vi "Process.vi"(8 "error in (no error)":errorcluster, 10 "Pound in":refnum<class "Pound.lvclass">, 11 "Qbus in":refnum<class "Qbus.lvclass">) -> (0 "error out":errorcluster)   [LabVIEW 2017, in "EmsaAnalysis.lvlib"]
uses:
  <vilib>/addons/InsightCM/Devices/Shared/Emsa/EmsaAnalysis/EmsaAnalysis.lvlib
  <vilib>/addons/Qbus/Qbus.lvclass
  <vilib>/NI/Software Watchdog/Pound/Pound.lvclass
  <vilib>/addons/InsightCM/Devices/Shared/Emsa/EmsaAnalysis/controls/datagroupMetrics.ctl
  <vilib>/addons/InsightCM/Devices/Shared/Emsa/EmsaAnalysis/controls/channelMetrics.ctl
  <vilib>/addons/InsightCM/Devices/Shared/Emsa/EmsaAnalysis/controls/metric.ctl
  <vilib>/addons/InsightCM/MessageBus/Base/controls/MetricDefinitionInstance.ctl
  <vilib>/addons/InsightCM/MessageBus/Base/controls/KeyValuePair.ctl
  <vilib>/addons/InsightCM/Devices/Shared/Emsa/EmsaAnalysis/controls/sweepInfo.ctl
  <vilib>/NI/Software Watchdog/Watchdog/Watchdog.lvclass
  <vilib>/addons/InsightCM/Devices/Shared/Common/DataFlow/DataFlow.lvlib
  <vilib>/addons/InsightCM/Devices/Shared/Common/DataEventCreator/DataEventCreator.lvlib
  <vilib>/addons/TraceLogger/TraceLogger.lvlib
  <vilib>/addons/InsightCM/Devices/Shared/Emsa/EmsaDataEventCreator/EmsaDataEventCreator.lvlib
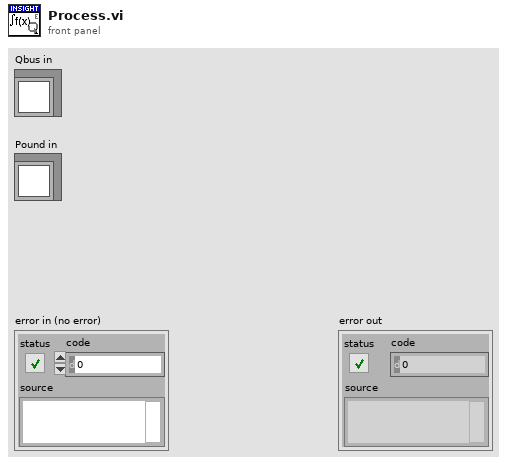
[diagram p1: front panel]
types:
  T1 = typedef "EmsaAnalysis.lvlib/datagroupMetrics.ctl" = cluster{"Name":string, "channels":T2[]}
  T2 = typedef "EmsaAnalysis.lvlib/channelMetrics.ctl" = cluster{"Name":string, "metrics":T3[], "sweeps":T6[]}
  T3 = typedef "EmsaAnalysis.lvlib/metric.ctl" = cluster{"TrendPointId":string, "ChannelId":string, "Metric Cfg":T4}
  T4 = typedef "MetricDefinitionInstance.ctl" = cluster{"Id":string, "MetricType":string, "Name":string, "Properties":T5[], "HighRate":bool}
  T5 = typedef "KeyValuePair.ctl" = cluster{"Key":string, "Value":string}
  T6 = typedef "EmsaAnalysis.lvlib/sweepInfo.ctl" = cluster{"start":dbl, "stop":dbl, "bandwidth":dbl}
  T7 = typedef "DataEventCreator.lvlib/RegisterTrendPoints.ctl" = cluster{"DataGroup":string, "Trends":T8[]}
  T8 = typedef "DataEventCreator.lvlib/Registry_Trend.ctl" = cluster{"TrendPointId":string, "DataSetName":string, "HighRate":bool, "Always Send":bool}
  T9 = typedef "DataFlow.lvlib/Data.ctl" = cluster{"DataGroup":string, "Waveforms":T10, "Map":T11, "Type":T12}
  T10 = typedef "wfmSGL_DVR.ctl" = refnum<data-value>
  T11 = typedef "PointValueMap.lvlib/PointMap.ctl" = refnum<data-value>
  T12 = typedef "DataFlow.lvlib/Type.ctl" = enum16{"High Rate", "Low Rate", "Burst Mode"}
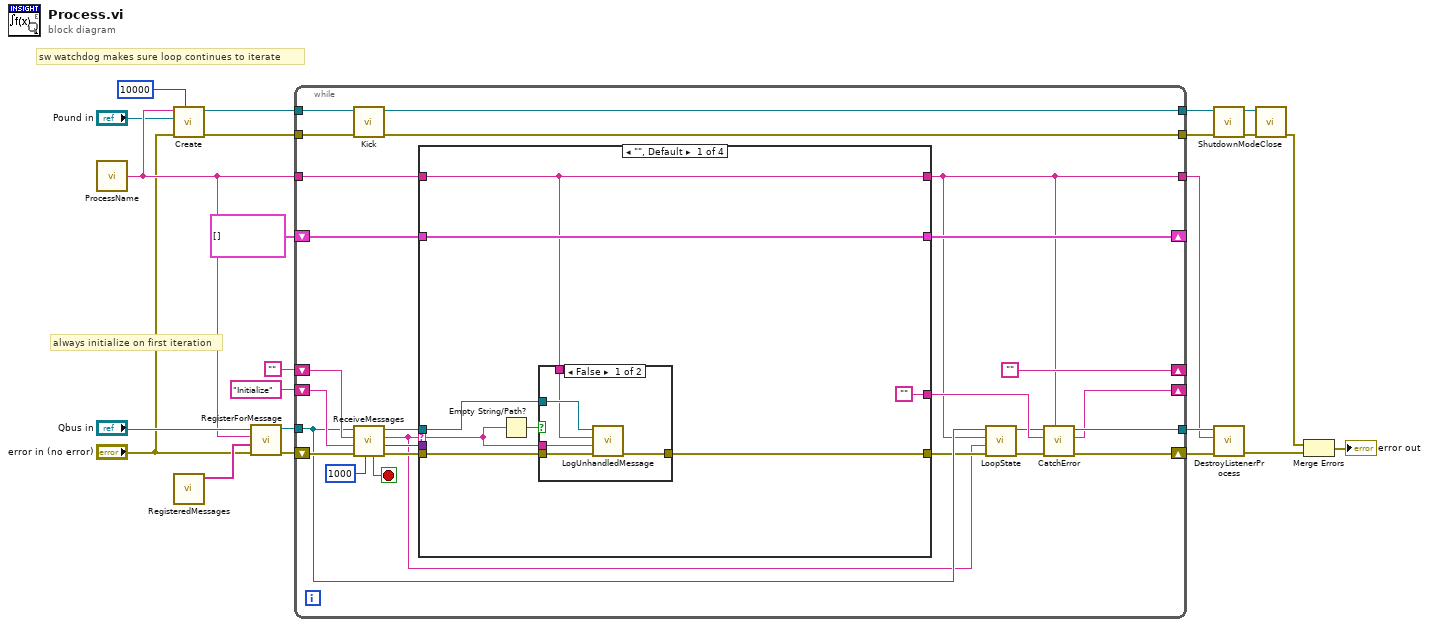
[diagram p0: block diagram]
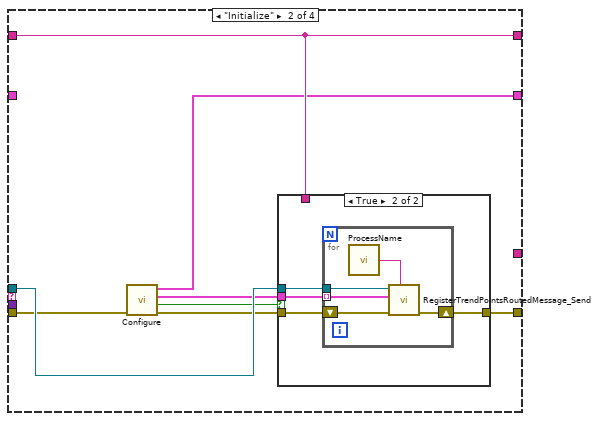
[diagram p3: hidden frame]
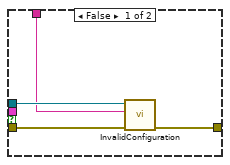
[diagram p4: hidden frame]
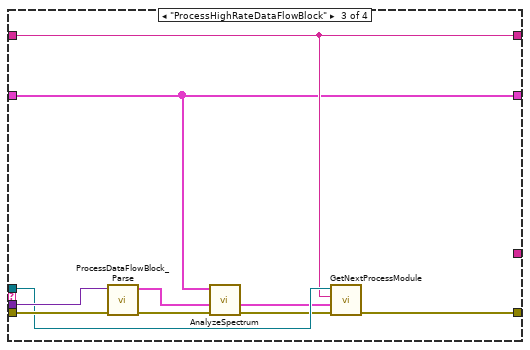
[diagram p5: hidden frame]
diagram:
  # "always initialize on first iteration"
  # "sw watchdog makes sure loop continues to iterate"
  n1 = call <vilib>:"ProcessName.vi"() -> ("process name"=w14:string)  [unwired: 5 in]
  n2 = call <vilib>:"Create.vi"("Execution Timeout (ms)"=u32 10000, "error in (no error)"="error in (no error)", "Pound"="Pound in", "Name"=w14) -> ("error out"=w7:errorcluster, "Watchdog"=w13:refnum<data-value>)  [unwired: 6 in]
  n3 = call <vilib>:"RegisteredMessages.vi"() -> ("registered messages"=w15:string[])  [unwired: 11 in]
  n4 = call <vilib>:"RegisterForMessage.vi"("error in (no error)"="error in (no error)", "message names"=w15, "process name"=w14, "Qbus in"="Qbus in") -> ("error in (no error)"=w22:errorcluster, "Qbus out"=w21:refnum<class "Qbus.lvclass">)  [unwired: 6 in]
  n5 = while {
    shift-right: [""] -> _
    shift-left: "" -> [w48]
    tunnel: w21 -> [w29]
    tunnel: w14 -> [w31]
    tunnel: [w39] -> w19
    tunnel: [w25] -> w18
    shift-right: [w38] -> _
    shift-left: "Initialize" -> [w43]
    shift-right: [w41] -> _
    shift-left: T1[] [] ("config") -> [w42]
    tunnel: w13 -> [w37]
    tunnel: [w36] -> w9
    tunnel: w7 -> [w35]
    tunnel: [w33] -> w6
    shift-right: [w40] -> w20
    shift-left: w22 -> [w34]
    stop <- w49 stop-if-true
    n6 = call <vilib>:"Kick.vi"("error in (no error)"=w35, "Watchdog"=w37) -> ("error out"=w33:errorcluster, "Watchdog"=w36:refnum<data-value>)  [unwired: 8 in]
    n7 = call <vilib>:"ReceiveMessages.vi"("Timeout(1000)"=1000 ("milliseconds to wait"), "error in (no error)"=w34, "priority action"=w43, "default action"=w48, "Qbus in"=w29) -> ("error out"=w47:errorcluster, "message value"=w44:variant, "action"=w24:string, "Qbus out"=w45:refnum<class "Qbus.lvclass">, "exit"=w49:bool)  [unwired: 2 in]
    n8 = case shown="\"\", Default" w24 {
      selector: w24 -> [w54 _ _ _]
      tunnel: w47 -> [w56 w68 w94 w97]
      tunnel: w45 -> [w52 w70 w91 _]
      tunnel: [w55 w71 w93 w97] -> w26
      tunnel: w44 -> [_ _ w92 _]
      tunnel: w42 -> [w57 _ w88 w96]
      tunnel: [w57 w66 w88 w96] -> w41
      tunnel: [w50 w69 w90 w95] -> w25
      tunnel: w31 -> [w50 w69 w90 w95]
      tunnel: ["" _ _ _] -> w30
      frame "", Default {
        n9 = Empty String/Path?(string/path=w54) -> (empty?=w53:bool)
        n10 = case shown="False" w53 {
          tunnel: [w58 w63] -> w55
          tunnel: w56 -> [w62 w63]
          tunnel: w54 -> [w61 _]
          tunnel: w52 -> [w60 _]
          tunnel: w50 -> [w59 _]
          frame False {
            n11 = call <vilib>:"LogUnhandledMessage.vi"("error in (no error)"=w62, "message"=w61, "process"=w59, "Qbus in"=w60) -> ("error out"=w58:errorcluster)  [unwired: 7 in]
          }
          frame True {
          }
        }
      }
      frame "Initialize" {
        n12 = call <vilib>:"Configure.vi"("error in (no error)"=w68) -> ("error out"=w67:errorcluster, "valid config"=w64:bool, "register trends"=w65:T7[], "config"=w66:T1[])  [unwired: 7 in]
        n13 = case shown="True" w64 {
          tunnel: w70 -> [w75 w77]
          tunnel: w65 -> [_ w76]
          tunnel: w67 -> [w74 w79]
          tunnel: [w73 w78] -> w71
          tunnel: w69 -> [w72 _]
          frame False {
            n14 = call <vilib>:"InvalidConfiguration.vi"("error in (no error)"=w74, "description"=w72, "Qbus in"=w75) -> ("error out"=w73:errorcluster)  [unwired: 7 in, 1 out]
          }
          frame True {
            n15 = for {
              shift-right: [w83] -> w78
              shift-left: w79 -> [w84]
              tunnel: w76 -> [w81] mode=indexing
              tunnel: w77 -> [w82]
              n16 = call <vilib>:"ProcessName.vi"() -> ("process name"=w80:string)  [unwired: 5 in]
              n17 = call <vilib>:"RegisterTrendPointsRoutedMessage_Send.vi"("data event creator process name"=w80, "error in (no error)"=w84, "register trend"=w81, "Qbus in"=w82) -> ("error out"=w83:errorcluster)  [unwired: 6 in, 1 out]
            }
          }
        }
      }
      frame "ProcessHighRateDataFlowBlock" {
        n18 = call <vilib>:"ProcessDataFlowBlock_Parse.vi"("error in (no error)"=w94, "body"=w92) -> ("error out"=w89:errorcluster, "data"=w87:T9)  [unwired: 8 in]
        n19 = call <vilib>:"AnalyzeSpectrum.vi"("error in (no error)"=w89, "data"=w87, "config"=w88) -> ("error out"=w85:errorcluster, "data out"=w86:T9)  [unwired: 7 in]
        n20 = call <vilib>:"GetNextProcessModule.vi"("error in (no error)"=w85, "data"=w86, "source"=w90, "Qbus in"=w91) -> ("error out"=w93:errorcluster)  [unwired: 6 in, 1 out]
      }
      frame "Exit" {
      }
    }
    n21 = call <vilib>:"LoopState.vi"("error in (no error)"=w26, "loop action"=w24, "process name"=w25, "Qbus in"=w29) -> ("error out"=w27:errorcluster, "Qbus out"=w28:refnum<class "Qbus.lvclass">)  [unwired: 6 in]
    n22 = call <vilib>:"CatchError.vi"("source"=w25, "error in (no error)"=w27, "next action in"=w30, "Qbus in"=w28) -> ("error out"=w40:errorcluster, "next action out"=w38:string, "Qbus out"=w39:refnum<class "Qbus.lvclass">)  [unwired: 5 in]
  }
  n23 = call <vilib>:"ShutdownMode.vi"("error in (no error)"=w6, "Watchdog"=w9) -> ("error out"=w8:errorcluster, "Watchdog"=w10:refnum<data-value>)  [unwired: 8 in]
  n24 = call <vilib>:"DestroyListenerProcess.vi"("error in (no error)"=w20, "process name"=w18, "Qbus in"=w19) -> ("error in (no error)"=w5:errorcluster)  [unwired: 7 in, 1 out]
  n25 = call <vilib>:"Close.vi"("error in (no error)"=w8, "Watchdog"=w10) -> ("error out"=w4:errorcluster)  [unwired: 9 in]
  n26 = Merge Errors(w4, w5) -> (→"error out":errorcluster)
